vi "ProtocolAnalysis.vi"(0 "TCP ref in":refnum<k5>, 11 "error in":errorcluster caption="错误输入") -> (4 "TCP ref out":refnum<k5>, 6 "Exit":bool, 15 "error out":errorcluster caption="错误输出")   [LabVIEW 2014]
uses:
  DataBase/DataBase.lvlib
  CYY/cyy.lvlib
panel:
  out "计数":i32
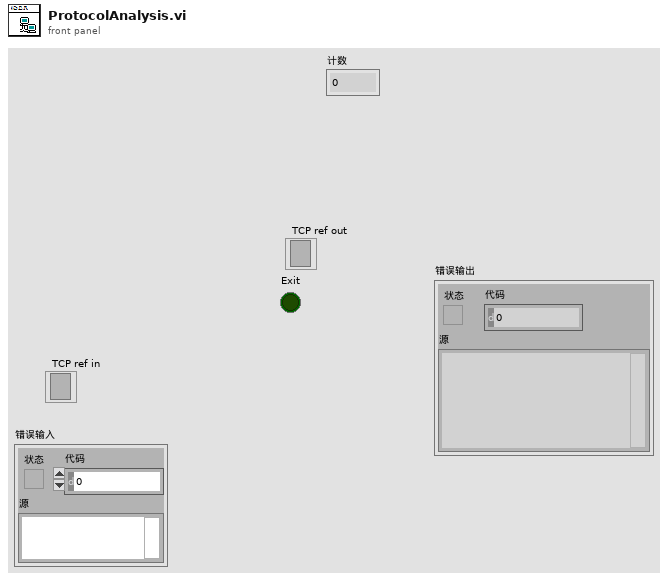
[diagram p1: front panel]
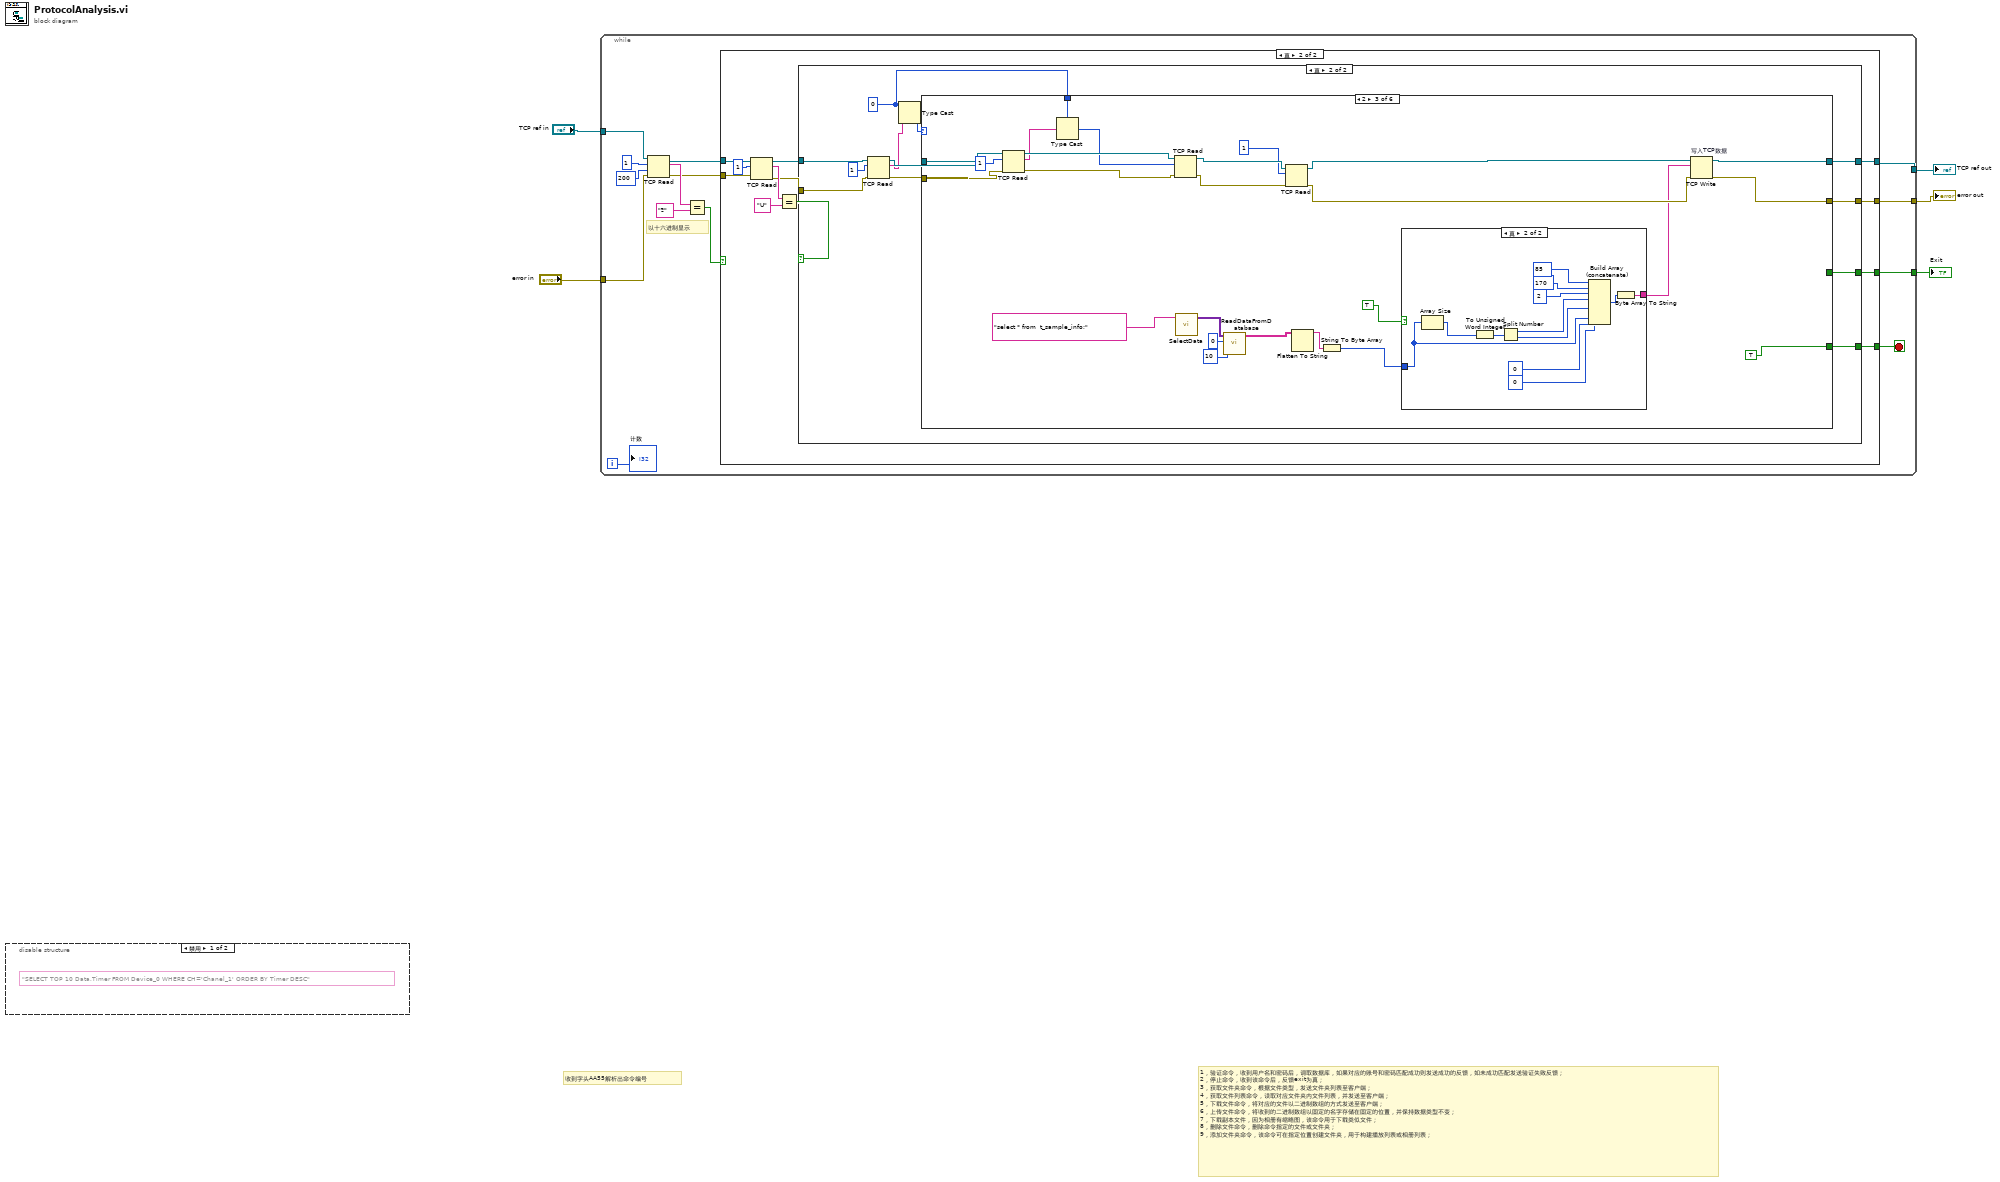
[diagram p0: block diagram]
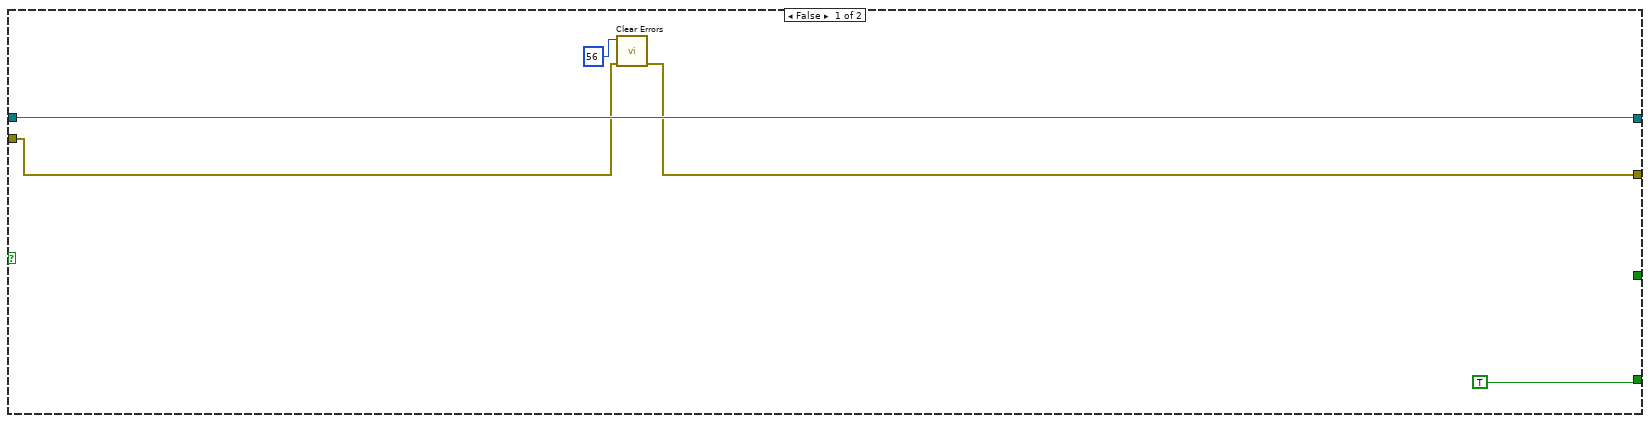
[diagram p2: hidden frame]
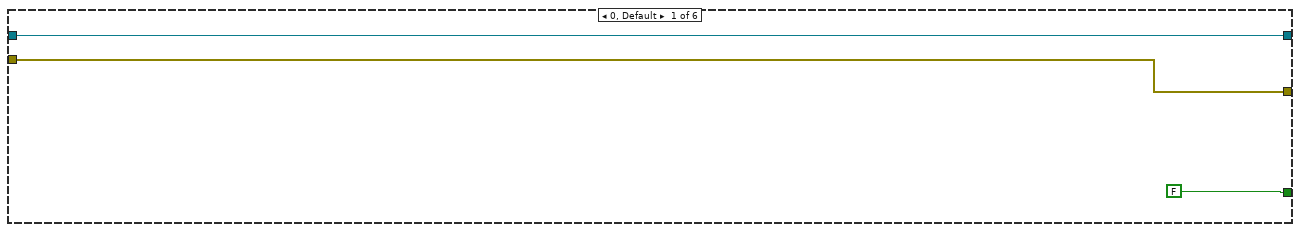
[diagram p4: hidden frame]
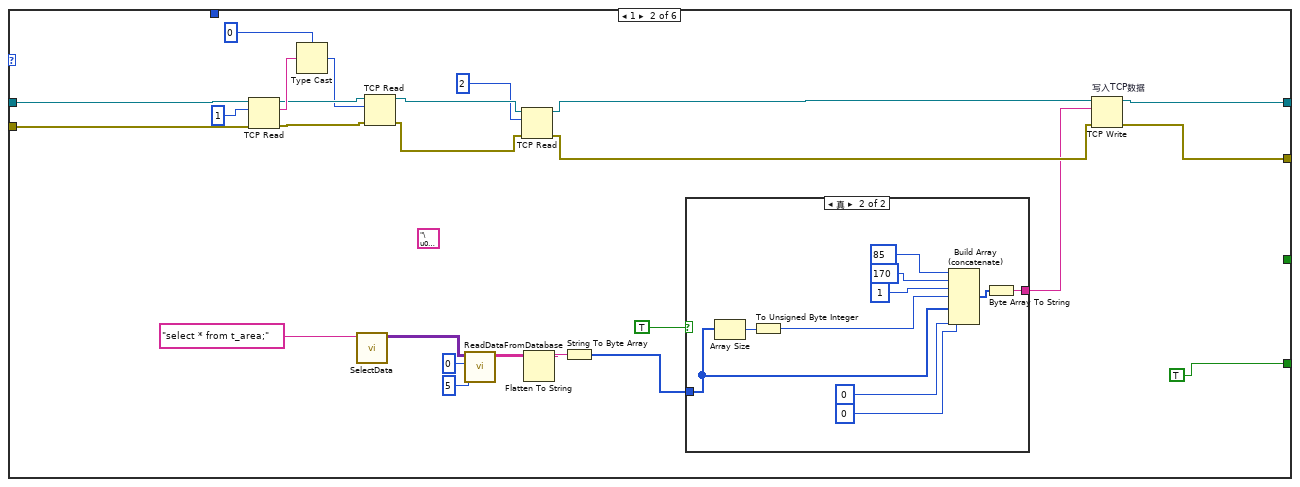
[diagram p5: hidden frame]
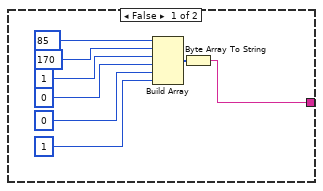
[diagram p6: hidden frame]
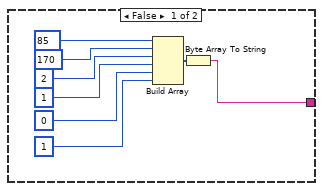
[diagram p7: hidden frame]
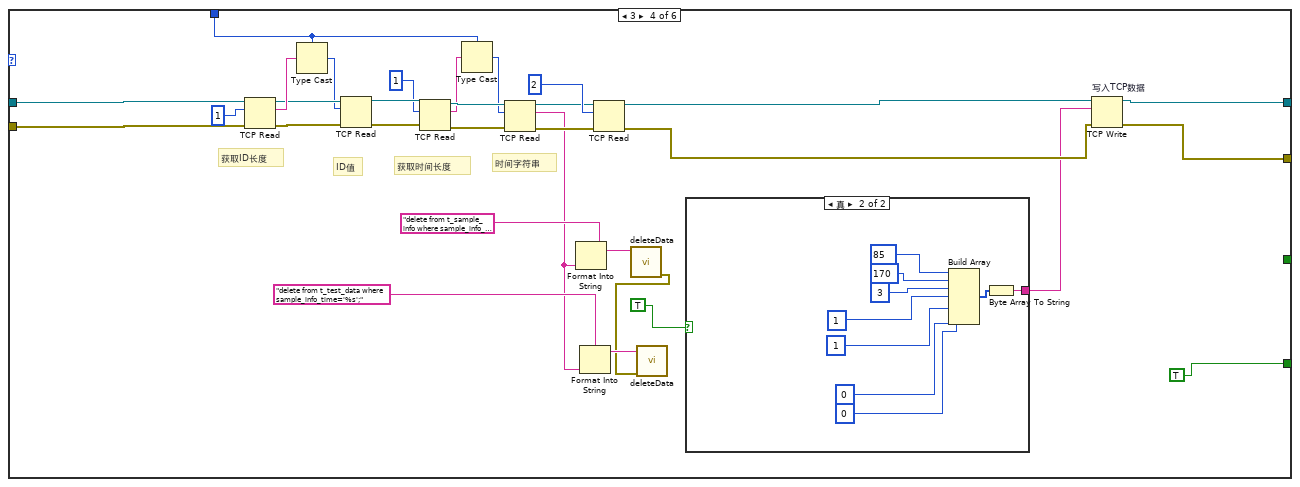
[diagram p8: hidden frame]
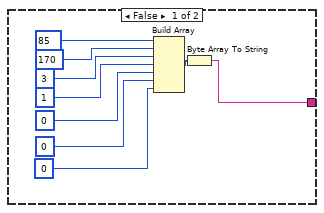
[diagram p9: hidden frame]
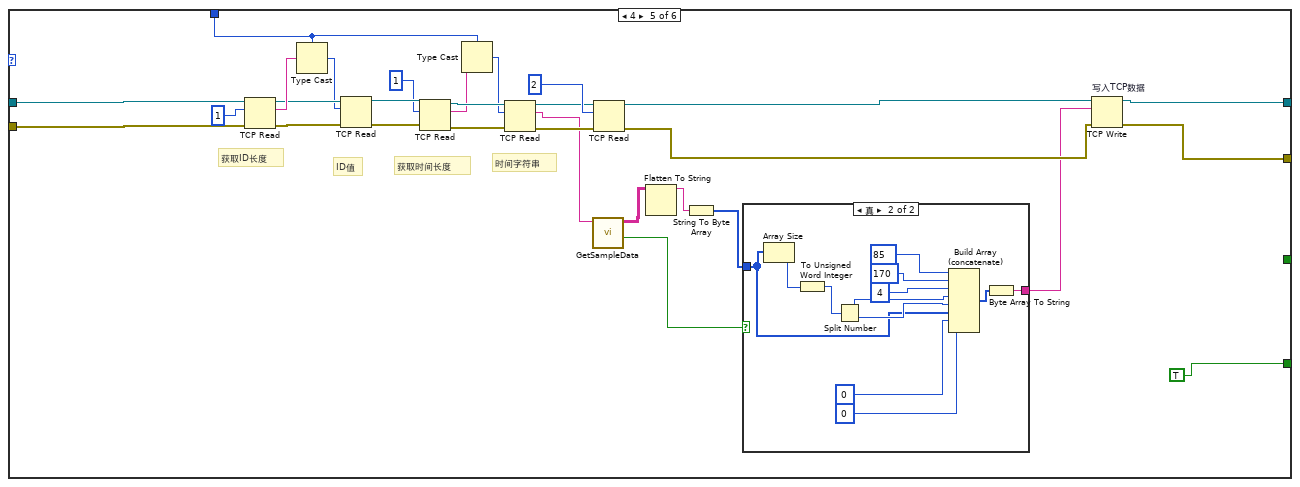
[diagram p10: hidden frame]
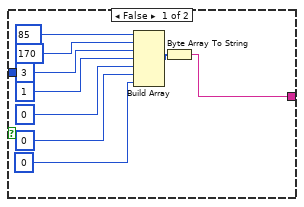
[diagram p11: hidden frame]
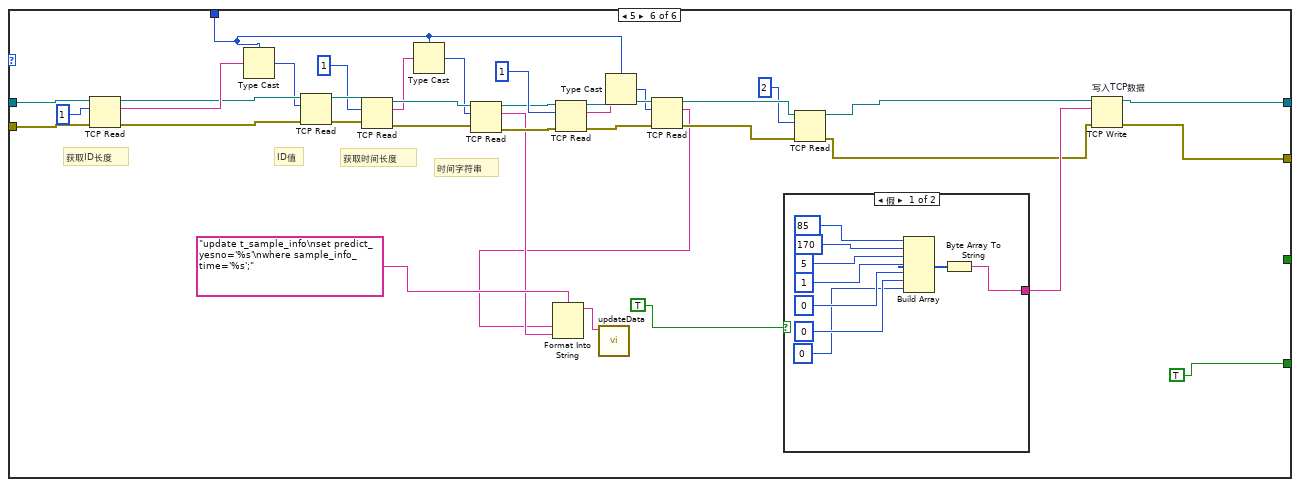
[diagram p12: hidden frame]
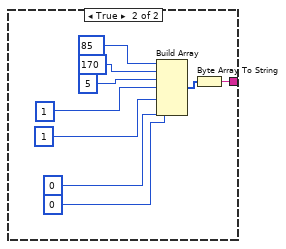
[diagram p13: hidden frame]
diagram:
  # "1，验证命令，收到用户名和密码后，调取数据库，如果对应的账号和密码匹配成功则发送成功的反馈，如未成功匹配发送验证失败反馈；\n2，停止命令，收到该命令后，反馈exit为真；\n3，获取文件夹命令，根据文件类型，发送文件夹列表至客户端；\n4，获取文件列表命令，读取对应文件夹内文件列表，并发送至客户端；\n5，下载文件命令，将对应的文件以二进制数组的方式发送至客户端；\n6，上传文件命令，将收到的二进制数组以固定的名字存储在固定的位置，并保持数据类型不变；\n7，下载副本文件，因为相册有缩略图，该命令用于下载类似文件；\n8，删除文件命令，删除命令指定的文件或文件夹；\n9，添加文件夹命令，该命令可在指定位置创建文件夹，用于构建播放列表或相册列表；"
  # "收到字头AA55解析出命令编号"
  n1 = disable-structure shown="禁用" {
    frame Disabled {
      (unwired) "SELECT TOP 10 Data,Timer FROM Device_0 WHERE CH='Chanel_1' ORDER BY Timer DESC" ("SQL query")
    }
    frame Enabled {
    }
  }
  n2 = while {
    tunnel: "TCP ref in" -> [w19]
    tunnel: "error in" -> [w18]
    tunnel: [w10] -> w3
    tunnel: [w9] -> w2
    tunnel: [w7] -> w1
    i -> [w6]
    stop <- w8 stop-if-true
    # "以十六进制显示"
    n3 = TCP Read(connection ID=w19, bytes to read=1 ("读取的字节"), error in (no error)=w18, 9:200 ("超时毫秒(25000)")) -> (connection ID out=w12:refnum<k5>, data out=w15:string, error out=w11:errorcluster)  [unwired: 1 in]
    n4 = Equal?(x=w15, y="ª") -> (x = y?=w13:bool)
    n5 = case shown="真" w13 {
      tunnel: w12 -> [w24 w33]
      tunnel: w11 -> [w22 w32]
      tunnel: [w24 w28] -> w10
      tunnel: [w21 w27] -> w9
      tunnel: [TRUE w26] -> w8
      tunnel: [_ w25] -> w7
      frame False {
        n6 = call <vilib>:"Clear Errors.vi"("error in (no error)"=w22, "specific error code to clear (0: all)"=56) -> ("error out"=w21:errorcluster)  [unwired: 4 in, 1 out]
      }
      frame True {
        n7 = TCP Read(connection ID=w33, bytes to read=1 ("读取的字节"), error in (no error)=w32) -> (connection ID out=w29:refnum<k5>, data out=w35:string, error out=w30:errorcluster)  [unwired: 2 in]
        n8 = Equal?(x=w35, y="U") -> (x = y?=w31:bool)
        n9 = case shown="真" w31 {
          tunnel: w30 -> [w37 w49]
          tunnel: w29 -> [w38 w48]
          tunnel: [w38 w46] -> w28
          tunnel: [w37 w45] -> w27
          tunnel: [_ w43] -> w26
          tunnel: [_ w42] -> w25
          frame False {
          }
          frame True {
            w39 = u8 0
            n10 = TCP Read(connection ID=w48, bytes to read=1 ("读取的字节"), error in (no error)=w49) -> (connection ID out=w47:refnum<k5>, data out=w41:string, error out=w44:errorcluster)  [unwired: 2 in]
            n11 = Type Cast(type=w39, x=w41) -> (*(type *) &x=w40:u8)
            n12 = case shown="2" w40 {
              tunnel: w47 -> [w53 w74 w118 w168 w215 w272]
              tunnel: [w53 w78 w121 w172 w219 w276] -> w46
              tunnel: [w52 w77 w107 w171 w218 w275] -> w45
              tunnel: w44 -> [w52 w73 w106 w167 w214 w271]
              tunnel: [_ TRUE TRUE TRUE TRUE TRUE] -> w43
              tunnel: [FALSE _ _ _ _ _] -> w42
              tunnel: w39 -> [_ _ w104 w144 w192 w242]
              frame 0, Default {
              }
              frame 1 {
                (unwired) "\u0000"
                n13 = TCP Read(connection ID=w74, bytes to read=1 ("读取的字节"), error in (no error)=w73) -> (connection ID out=w71:refnum<k5>, data out=w72:string, error out=w68:errorcluster)  [unwired: 2 in]
                n14 = Type Cast(type=u8 0, x=w72) -> (*(type *) &x=w54:u8)
                n15 = call "SelectData.vi"("SQL query"="select * from t_area;") -> ("recordset data"=w61:variant[][])  [unwired: 7 in, 1 out]
                n16 = TCP Read(connection ID=w71, bytes to read=w54, error in (no error)=w68) -> (connection ID out=w70:refnum<k5>, error out=w67:errorcluster)  [unwired: 2 in, 1 out]
                n17 = call "ReadDataFromDatabase.vi"("长度"=5, "index"=0, "recordset data"=w61) -> ("所有记录"=w57:string[][])  [unwired: 7 in, 1 out]
                n18 = TCP Read(connection ID=w70, bytes to read=2, error in (no error)=w67) -> (connection ID out=w69:refnum<k5>, error out=w66:errorcluster)  [unwired: 2 in, 1 out]
                n19 = Flatten To String(anything=w57) -> (data string=w58:string)  [unwired: 3 in, 2 out]
                n20 = String To Byte Array(string=w58) -> (unsigned byte array=w64:u8[])
                n21 = case shown="真" TRUE {
                  tunnel: w64 -> [_ w90]
                  tunnel: [w79 w89] -> w63
                  frame False {
                    n22 = Build Array(u8 85, u8 170, u8 1, u8 0, u8 0, u8 1) -> (w80:u8[])
                    n23 = Byte Array To String(unsigned byte array=w80) -> (string=w79:string)
                  }
                  frame True {
                    n24 = Array Size(array=w90) -> (size(s)=w92:i32)
                    n25 = To Unsigned Byte Integer(number=w92) -> (unsigned 8bit integer=w91:u8)
                    n26 = Build Array (concatenate)(u8 85, u8 170, u8 1, w91, w90, u8 0, u8 0) -> (w93:u8[])
                    n27 = Byte Array To String(unsigned byte array=w93) -> (string=w89:string)
                  }
                }
                n28 = TCP Write "写入TCP数据"(connection ID=w69, data in=w63, error in (no error)=w66) -> (connection ID out=w78:refnum<k5>, error out=w77:errorcluster)  [unwired: 1 in, 1 out]
              }
              frame 2 {
                n29 = TCP Read(connection ID=w118, bytes to read=1 ("读取的字节"), error in (no error)=w106) -> (connection ID out=w117:refnum<k5>, data out=w105:string, error out=w114:errorcluster)  [unwired: 2 in]
                n30 = Type Cast(type=w104, x=w105) -> (*(type *) &x=w103:u8)
                n31 = TCP Read(connection ID=w117, bytes to read=w103, error in (no error)=w114) -> (connection ID out=w116:refnum<k5>, error out=w113:errorcluster)  [unwired: 2 in, 1 out]
                n32 = call "SelectData.vi"("SQL query"="select * from  t_sample_info;") -> ("recordset data"=w102:variant[][])  [unwired: 7 in, 1 out]
                n33 = call "ReadDataFromDatabase.vi"("长度"=10, "index"=0, "recordset data"=w102) -> ("所有记录"=w97:string[][])  [unwired: 7 in, 1 out]
                n34 = TCP Read(connection ID=w116, bytes to read=1, error in (no error)=w113) -> (connection ID out=w115:refnum<k5>, error out=w112:errorcluster)  [unwired: 2 in, 1 out]
                n35 = Flatten To String(anything=w97) -> (data string=w99:string)  [unwired: 3 in, 2 out]
                n36 = String To Byte Array(string=w99) -> (unsigned byte array=w110:u8[])
                n37 = case shown="真" TRUE {
                  tunnel: w110 -> [_ w132]
                  tunnel: [w122 w137] -> w109
                  frame False {
                    n38 = Build Array(u8 85, u8 170, u8 2, u8 1, u8 0, u8 1) -> (w123:u8[])
                    n39 = Byte Array To String(unsigned byte array=w123) -> (string=w122:string)
                  }
                  frame True {
                    n40 = Array Size(array=w132) -> (size(s)=w135:i32)
                    n41 = To Unsigned Word Integer(number=w135) -> (unsigned 16bit integer=w136:u16)
                    n42 = Split Number(x=w136) -> (hi(x)=w134:u8, lo(x)=w133:u8)
                    n43 = Build Array (concatenate)(u8 85, u8 170, u8 2, w134, w133, w132, u8 0, u8 0) -> (w138:u8[])
                    n44 = Byte Array To String(unsigned byte array=w138) -> (string=w137:string)
                  }
                }
                n45 = TCP Write "写入TCP数据"(connection ID=w115, data in=w109, error in (no error)=w112) -> (connection ID out=w121:refnum<k5>, error out=w107:errorcluster)  [unwired: 1 in, 1 out]
              }
              frame 3 {
                # "时间字符串"
                # "获取时间长度"
                # "ID值"
                # "获取ID长度"
                n46 = TCP Read(connection ID=w168, bytes to read=1 ("读取的字节"), error in (no error)=w167) -> (connection ID out=w165:refnum<k5>, data out=w166:string, error out=w163:errorcluster)  [unwired: 2 in]
                n47 = Type Cast(type=w144, x=w166) -> (*(type *) &x=w143:u8)
                n48 = TCP Read(connection ID=w165, bytes to read=w143, error in (no error)=w163) -> (connection ID out=w158:refnum<k5>, error out=w155:errorcluster)  [unwired: 2 in, 1 out]
                n49 = TCP Read(connection ID=w158, bytes to read=1, error in (no error)=w155) -> (connection ID out=w157:refnum<k5>, data out=w152:string, error out=w154:errorcluster)  [unwired: 2 in]
                n50 = Type Cast(type=w144, x=w152) -> (*(type *) &x=w142:u8)
                n51 = TCP Read(connection ID=w157, bytes to read=w142, error in (no error)=w154) -> (connection ID out=w156:refnum<k5>, data out=w147:string, error out=w153:errorcluster)  [unwired: 2 in]
                n52 = Format Into String(format string="delete from t_sample_info where sample_info_time='%s';", w147) -> (resulting string=w149:string)  [unwired: 2 in, 1 out]
                n53 = Format Into String(format string="delete from t_test_data where sample_info_time='%s';", w147) -> (resulting string=w146:string)  [unwired: 2 in, 1 out]
                n54 = TCP Read(connection ID=w156, bytes to read=2, error in (no error)=w153) -> (connection ID out=w164:refnum<k5>, error out=w162:errorcluster)  [unwired: 2 in, 1 out]
                n55 = call "deleteData.vi"("SQL query"=w149) -> ("error out"=w145:errorcluster)  [unwired: 10 in]
                n56 = call "deleteData.vi"("error in"=w145, "SQL query"=w146) -> ()  [unwired: 9 in, 1 out]
                n57 = case shown="真" TRUE {
                  tunnel: [w174 w186] -> w160
                  frame False {
                    n58 = Build Array(u8 85, u8 170, u8 3, u8 1, u8 0, u8 0, u8 0) -> (w175:u8[])
                    n59 = Byte Array To String(unsigned byte array=w175) -> (string=w174:string)
                  }
                  frame True {
                    n60 = Build Array(u8 85, u8 170, u8 3, u8 1, u8 1, u8 0, u8 0) -> (w187:u8[])
                    n61 = Byte Array To String(unsigned byte array=w187) -> (string=w186:string)
                  }
                }
                n62 = TCP Write "写入TCP数据"(connection ID=w164, data in=w160, error in (no error)=w162) -> (connection ID out=w172:refnum<k5>, error out=w171:errorcluster)  [unwired: 1 in, 1 out]
              }
              frame 4 {
                # "时间字符串"
                # "获取时间长度"
                # "ID值"
                # "获取ID长度"
                n63 = TCP Read(connection ID=w215, bytes to read=1 ("读取的字节"), error in (no error)=w214) -> (connection ID out=w212:refnum<k5>, data out=w213:string, error out=w210:errorcluster)  [unwired: 2 in]
                n64 = Type Cast(type=w192, x=w213) -> (*(type *) &x=w193:u8)
                n65 = TCP Read(connection ID=w212, bytes to read=w193, error in (no error)=w210) -> (connection ID out=w206:refnum<k5>, error out=w203:errorcluster)  [unwired: 2 in, 1 out]
                n66 = TCP Read(connection ID=w206, bytes to read=1, error in (no error)=w203) -> (connection ID out=w205:refnum<k5>, data out=w200:string, error out=w202:errorcluster)  [unwired: 2 in]
                n67 = Type Cast(type=w192, x=w200) -> (*(type *) &x=w191:u8)
                n68 = TCP Read(connection ID=w205, bytes to read=w191, error in (no error)=w202) -> (connection ID out=w204:refnum<k5>, data out=w198:string, error out=w201:errorcluster)  [unwired: 2 in]
                n69 = call "GetSampleData.vi"("SampleInfoTime"=w198) -> ("是否存在记录"=w197:bool, "所有记录"=w195:string[][])  [unwired: 7 in, 2 out]
                n70 = TCP Read(connection ID=w204, bytes to read=2, error in (no error)=w201) -> (connection ID out=w211:refnum<k5>, error out=w209:errorcluster)  [unwired: 2 in, 1 out]
                n71 = Flatten To String(anything=w195) -> (data string=w196:string)  [unwired: 3 in, 2 out]
                n72 = String To Byte Array(string=w196) -> (unsigned byte array=w194:u8[])
                n73 = case shown="真" w197 {
                  tunnel: [w221 w236] -> w207
                  tunnel: w194 -> [_ w231]
                  frame False {
                    n74 = Build Array(u8 85, u8 170, u8 3, u8 1, u8 0, u8 0, u8 0) -> (w222:u8[])
                    n75 = Byte Array To String(unsigned byte array=w222) -> (string=w221:string)
                  }
                  frame True {
                    n76 = Array Size(array=w231) -> (size(s)=w235:i32)
                    n77 = To Unsigned Word Integer(number=w235) -> (unsigned 16bit integer=w234:u16)
                    n78 = Split Number(x=w234) -> (hi(x)=w233:u8, lo(x)=w232:u8)
                    n79 = Build Array (concatenate)(u8 85, u8 170, u8 4, w233, w232, w231, u8 0, u8 0) -> (w237:u8[])
                    n80 = Byte Array To String(unsigned byte array=w237) -> (string=w236:string)
                  }
                }
                n81 = TCP Write "写入TCP数据"(connection ID=w211, data in=w207, error in (no error)=w209) -> (connection ID out=w219:refnum<k5>, error out=w218:errorcluster)  [unwired: 1 in, 1 out]
              }
              frame 5 {
                # "时间字符串"
                # "获取时间长度"
                # "ID值"
                # "获取ID长度"
                n82 = TCP Read(connection ID=w272, bytes to read=1 ("读取的字节"), error in (no error)=w271) -> (connection ID out=w269:refnum<k5>, data out=w270:string, error out=w268:errorcluster)  [unwired: 2 in]
                n83 = Type Cast(type=w242, x=w270) -> (*(type *) &x=w244:u8)
                n84 = TCP Read(connection ID=w269, bytes to read=w244, error in (no error)=w268) -> (connection ID out=w264:refnum<k5>, error out=w261:errorcluster)  [unwired: 2 in, 1 out]
                n85 = TCP Read(connection ID=w264, bytes to read=1, error in (no error)=w261) -> (connection ID out=w263:refnum<k5>, data out=w258:string, error out=w260:errorcluster)  [unwired: 2 in]
                n86 = Type Cast(type=w242, x=w258) -> (*(type *) &x=w243:u8)
                n87 = TCP Read(connection ID=w263, bytes to read=w243, error in (no error)=w260) -> (connection ID out=w262:refnum<k5>, data out=w247:string, error out=w259:errorcluster)  [unwired: 2 in]
                n88 = TCP Read(connection ID=w262, bytes to read=1, error in (no error)=w259) -> (connection ID out=w256:refnum<k5>, data out=w249:string, error out=w254:errorcluster)  [unwired: 2 in]
                n89 = Type Cast(type=w242, x=w249) -> (*(type *) &x=w241:u8)
                n90 = TCP Read(connection ID=w256, bytes to read=w241, error in (no error)=w254) -> (connection ID out=w252:refnum<k5>, data out=w246:string, error out=w255:errorcluster)  [unwired: 2 in]
                n91 = Format Into String(format string="update t_sample_info\nset predict_yesno='%s'\nwhere sample_info_time='%s';", w246, w247) -> (resulting string=w245:string)  [unwired: 2 in, 1 out]
                n92 = call "updateData.vi"("SQL query"=w245) -> ()  [unwired: 10 in, 1 out]
                n93 = case shown="假" TRUE {
                  tunnel: [w278 w290] -> w266
                  frame False {
                    n94 = Build Array(u8 85, u8 170, u8 5, u8 1, u8 0, u8 0, u8 0) -> (w279:u8[])
                    n95 = Byte Array To String(unsigned byte array=w279) -> (string=w278:string)
                  }
                  frame True {
                    n96 = Build Array(u8 85, u8 170, u8 5, u8 1, u8 1, u8 0, u8 0) -> (w291:u8[])
                    n97 = Byte Array To String(unsigned byte array=w291) -> (string=w290:string)
                  }
                }
                n98 = TCP Read(connection ID=w252, bytes to read=2, error in (no error)=w255) -> (connection ID out=w251:refnum<k5>, error out=w253:errorcluster)  [unwired: 2 in, 1 out]
                n99 = TCP Write "写入TCP数据"(connection ID=w251, data in=w266, error in (no error)=w253) -> (connection ID out=w276:refnum<k5>, error out=w275:errorcluster)  [unwired: 1 in, 1 out]
              }
            }
          }
        }
      }
    }
    "计数" <- w6
  }
  "error out" <- w2
  "TCP ref out" <- w3
  "Exit" <- w1
